vi "Unubscribe Request.vi"(6 "Broadcaster":string, 8 "error in (no error)":errorcluster, 9 "Subscriber Enqueuer":refnum<class "Message Enqueuer.lvclass">, 10 "Topic":string, 11 "Measure Object in":refnum<class "Template Module.lvclass">) -> (0 "error out":errorcluster, 3 "Measure Object out":refnum<class "Template Module.lvclass">)   [LabVIEW 2018, in "Template Module.lvclass"]
uses:
  Template Module.lvclass
  <vilib>/ActorFramework/Message Enqueuer/Message Enqueuer.lvclass
  Template Module.lvclass/Template Module.ctl
  Template Module Messages/Unubscribe Request Msg/Unubscribe Request Msg.lvclass/Unubscribe Request Msg.ctl
  <vilib>/ActorFramework/Message Enqueuer/Message Enqueuer.lvclass/Message Enqueuer.ctl
  Read Name.vi
  <vilib>/ActorFramework/Message Enqueuer/Enqueue.vi
  Template Module Messages/Unubscribe Request Msg/Unubscribe Request Msg.lvclass
  C:/Program Files/National Instruments/LabVIEW 2018/vi.lib/ActorFramework/Message/Message.lvclass
  <vilib>/ActorFramework/Message Priority Queue/Priority Enqueue.vi
  BroadcastBroker/BroadcastBroker.lvclass
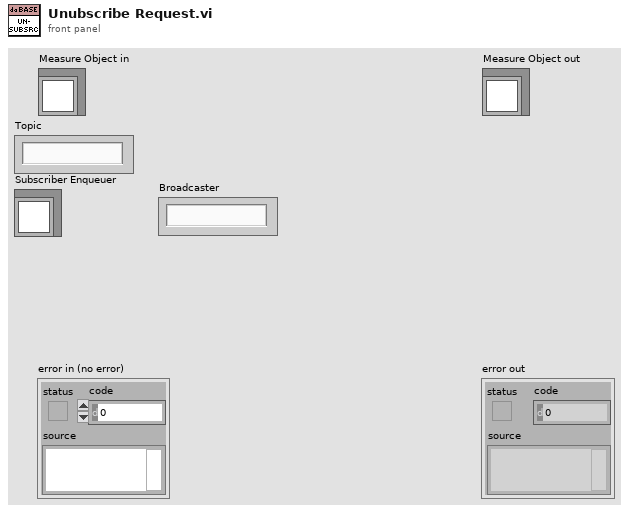
[diagram p1: front panel]
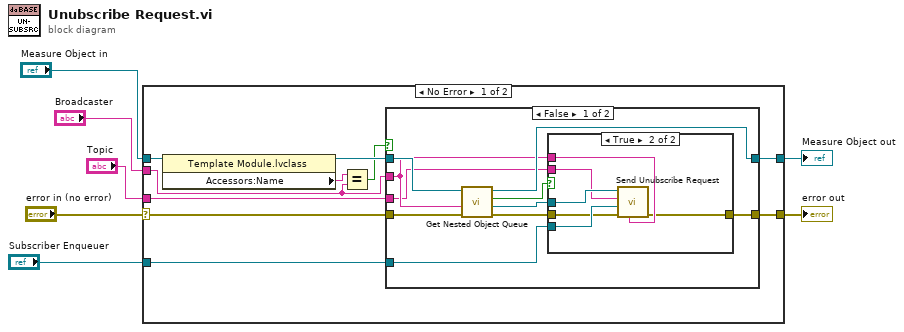
[diagram p0: block diagram]
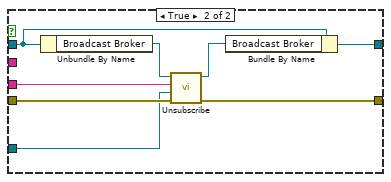
[diagram p3: hidden frame]
diagram:
  n1 = case shown="No Error" "error in (no error)" {
    selector: "error in (no error)" -> [w17 w44]
    tunnel: [w16 w44] -> w6
    tunnel: [w15 w43] -> w4
    tunnel: "Measure Object in" -> [w13 w43]
    tunnel: "Broadcaster" -> [w10 _]
    tunnel: "Topic" -> [w9 _]
    tunnel: "Subscriber Enqueuer" -> [w8 _]
    frame No Error {
      n2 = property class="Template Module.lvclass"(reference=w13) -> (reference out=w12:refnum<class "Template Module.lvclass">, "Accessors:Name"=w14:string)  [unwired: 1 in, 1 out]
      n3 = Equal?(x=w14, y=w10) -> (x = y?=w11:bool)
      n4 = case shown="False" w11 {
        tunnel: w12 -> [w21 w42]
        tunnel: w17 -> [w24 w40]
        tunnel: [w23 w39] -> w16
        tunnel: [w22 w38] -> w15
        tunnel: w10 -> [w20 _]
        tunnel: w9 -> [w19 w36]
        tunnel: w8 -> [w18 w35]
        frame False {
          n5 = call-dynamic "Get Nested Object Queue.vi"("error in (no error)"=w24, "Name"=w20, "Measure Object in"=w21) -> ("error out"=w27:errorcluster, "Object Enqueuer"=w26:refnum<class "Message Enqueuer.lvclass">, "Found?"=w25:bool, "Measure Object out"=w22:refnum<class "Template Module.lvclass">)  [unwired: 5 in]
          n6 = case shown="True" w25 {
            tunnel: w26 -> [_ w34]
            tunnel: w27 -> [w28 w30]
            tunnel: w20 -> [_ w31]
            tunnel: [w28 w29] -> w23
            tunnel: w18 -> [_ w33]
            tunnel: w19 -> [_ w32]
            frame False {
            }
            frame True {
              n7 = call "Send Unubscribe Request.vi"("Broadcaster"=w31, "error in (no error)"=w30, "Subscriber Enqueuer"=w33, "Topic"=w32, "Message Enqueuer"=w34) -> ("error out"=w29:errorcluster)  [unwired: 5 in, 1 out]
            }
          }
        }
        frame True {
          n8 = Unbundle By Name(w42) -> ("Broadcast Broker"=w41:refnum<class "BroadcastBroker.lvclass">)
          n9 = call-dynamic "Unsubscribe.vi"("error in (no error)"=w40, "Subscriber Enqueuer"=w35, "Topic"=w36, "Broadcaster in"=w41) -> ("error out"=w39:errorcluster, "Broadcaster out"=w37:refnum<class "BroadcastBroker.lvclass">)  [unwired: 6 in]
          n10 = Bundle By Name(cluster=w42, "Broadcast Broker"=w37) -> (w38:refnum<class "Template Module.lvclass">)
        }
      }
    }
    frame Error {
    }
  }
  "error out" <- w6
  "Measure Object out" <- w4
